vi "1D force plotting.vi"(0 "Calibration":u16(ring)=2 items=["None", "Position", "Force"], 1 "Forces":waveform(dbl)[](array[waveform]), 2 "Deflections":waveform(dbl)[](array[waveform]), 3 "Raw Data":waveform(dbl)[](array[waveform]), 4 "Only check fixed trap T2":bool) -> (5 "Vec Mean of T1 T2":dbl[](array[numeric])=[466.5641880718258, 401.4208374052827], 6 "Output force values":T1={"T1 X"=1434.5224195674728, "T2 X"=566.5373940903642, "Mean"=433.9925127385543, "Difference"=2001.059813657837} {"Difference" format="%.2g"; "Mean" format="%#_3g"; "T2 X" format="%0.2f"; "T1 X" format="%0.2f"}, 7 "Output waveforms":waveform(dbl)[](array[waveform]))   [LabVIEW 2014]
uses:
  <vilib>/Analysis/baseanly.llb/Mean (DBL).vi
  <vilib>/Analysis/NI_AALBase.lvlib
panel:
  in  "Force values":T1={"T1 X"=1434.5224195674728, "T2 X"=566.5373940903642, "Mean"=433.9925127385543, "Difference"=2001.059813657837} {"Difference" format="%.2g"; "Mean" format="%#_3g"; "T2 X" format="%0.2f"; "T1 X" format="%0.2f"}
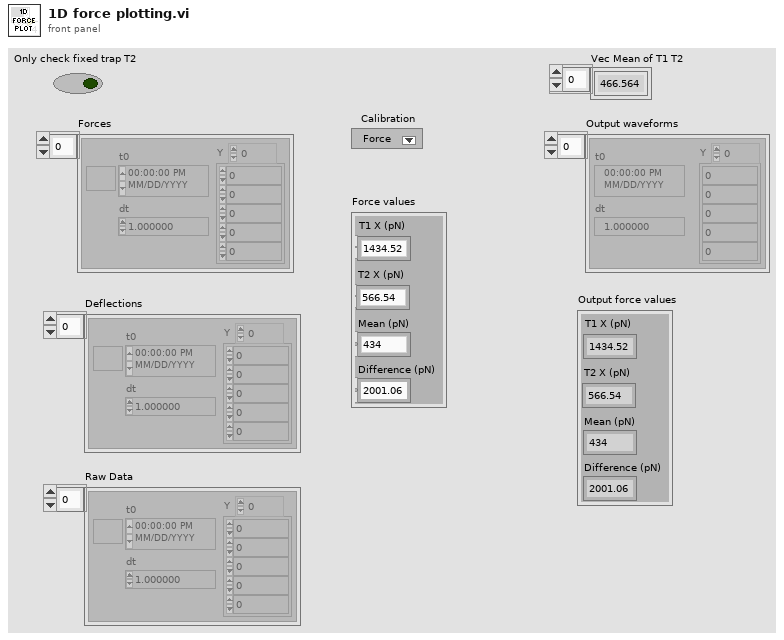
[diagram p1: front panel]
types:
  T1 = cluster{"T1 X":dbl, "T2 X":dbl, "Mean":dbl, "Difference":dbl}
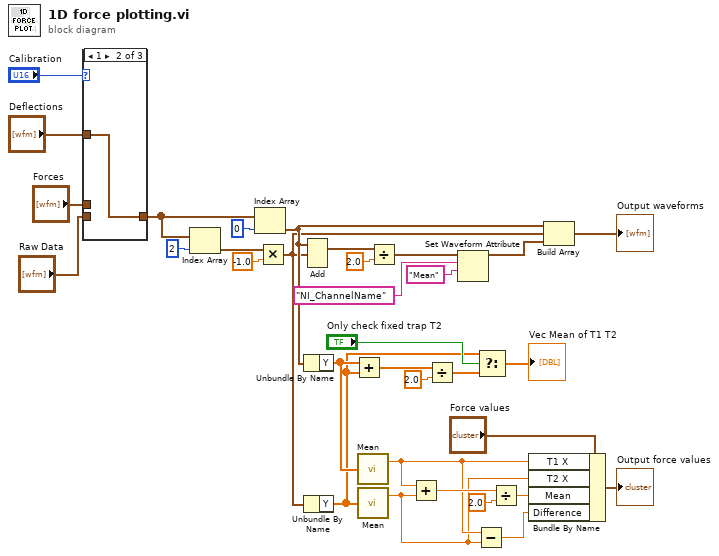
[diagram p0: block diagram]
diagram:
  n1 = case shown="1" "Calibration" {
    tunnel: "Forces" -> [_ _ w36]
    tunnel: [w34 w35 w36] -> w31
    tunnel: "Deflections" -> [_ w35 _]
    tunnel: "Raw Data" -> [w34 _ _]
    frame 0, Default {
    }
    frame 1 {
    }
    frame 2 {
    }
  }
  n2 = Index Array(array=w31, index=2) -> (element=w23:waveform(dbl))
  n3 = Index Array(array=w31, index=0) -> (element=w22:waveform(dbl))
  n4 = Multiply(x=w23, y=-1.0) -> (x*y=w21:waveform(dbl))
  n5 = Add(1:w21, 2:w22) -> (0:w25:waveform(dbl))  [unwired: 1 in, 1 out]
  n6 = Unbundle By Name(w22) -> ("Y"=w13:dbl[])
  n7 = Unbundle By Name(w21) -> ("Y"=w8:dbl[])
  n8 = Add(x=w13, y=w8) -> (x+y=w11:dbl[])
  n9 = call-poly <vilib>:"Mean.vi"("X"=w13) -> ("mean"=w16:dbl)  [unwired: 1 out]
  n10 = call-poly <vilib>:"Mean.vi"("X"=w8) -> ("mean"=w15:dbl)  [unwired: 1 out]
  n11 = Divide(x=w25, y=2.0) -> (x/y=w4:waveform(dbl))
  n12 = Add(x=w16, y=w15) -> (x+y=w18:dbl)
  n13 = Divide(x=w11, y=2.0) -> (x/y=w9:dbl[])
  n14 = Set Waveform Attribute(5:"Mean", 6:"NI_ChannelName", 7:w4) -> (3:w3:waveform(dbl))  [unwired: 1 in, 2 out]
  n15 = Subtract(x=w16, y=w15) -> (x-y=w14:dbl)
  n16 = Select(t=w8, s="Only check fixed trap T2", f=w9) -> (s? t:f=→"Vec Mean of T1 T2":dbl[])
  n17 = Divide(x=w18, y=2.0) -> (x/y=w17:dbl)
  n18 = Bundle By Name(cluster="Force values", "T1 X"=w16, "T2 X"=w15, "Mean"=w17, "Difference"=w14) -> (→"Output force values":T1)
  n19 = Build Array(w22, w21, w3) -> (→"Output waveforms":waveform(dbl)[])
